vi "Read AppInst.vi"(11 "Message Maker in":refnum<class "Message Scripter.lvclass">) -> (2 "AppInst":refnum<vi>)   [LabVIEW 2020, in "Message Maker.lvlib" / "Message Scripter.lvclass"]
uses:
  Message Scripter.lvclass
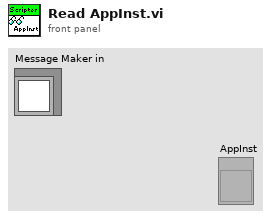
[diagram p1: front panel]
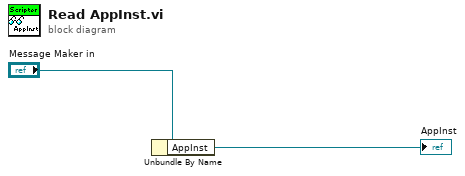
[diagram p0: block diagram]
diagram:
  n1 = Unbundle By Name("Message Maker in") -> ("AppInst"=→"AppInst":refnum<vi>)
